vi "liveCameraView.vi"(1 "Data 16":u16[][](array[numeric])) -> (0 "VI Refnum":refnum<vi>)   [LabVIEW 2015]
panel:
  out "Image display":u16[][](graph)
  in  "Close window":bool
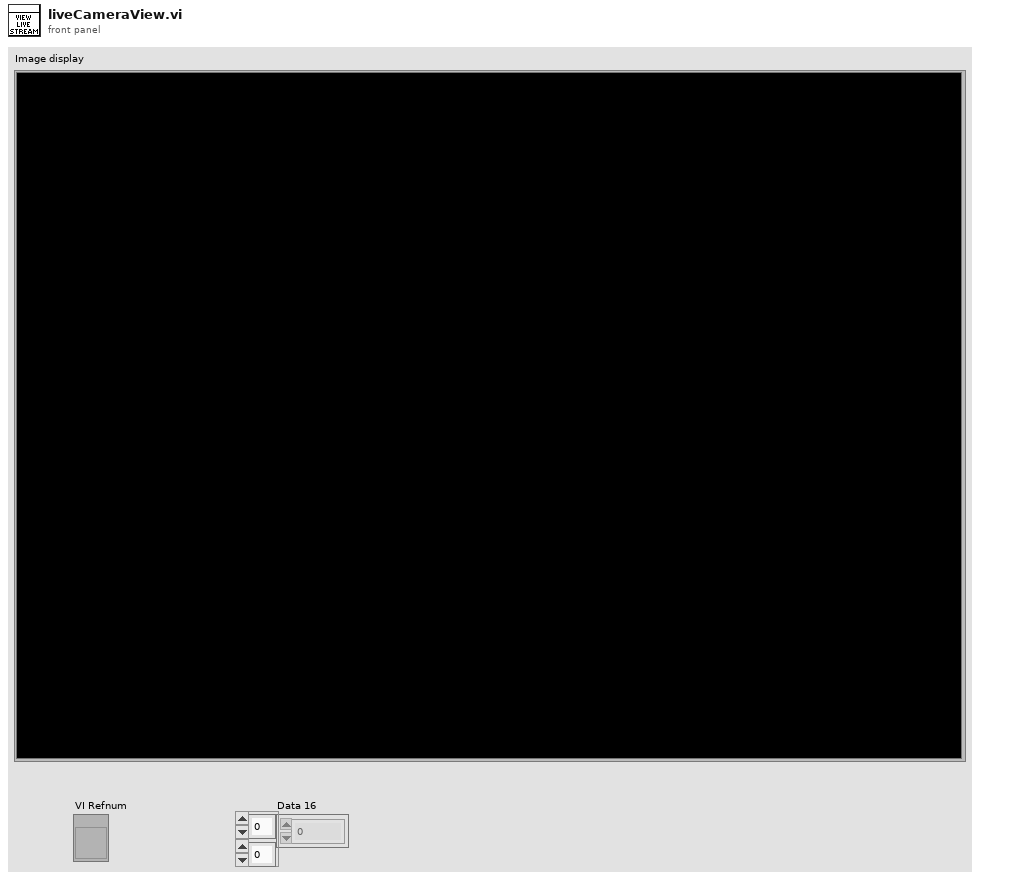
[diagram p1: front panel]
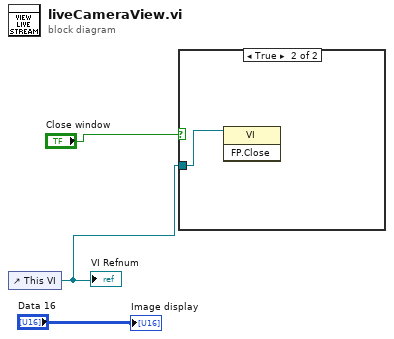
[diagram p0: block diagram]
diagram:
  n1 = control-ref of="This VI"() -> (w2:refnum<vi>)
  "VI Refnum" <- w2
  n2 = case shown="True" "Close window" {
    tunnel: w2 -> [_ w4]
    frame False {
    }
    frame True {
      n3 = invoke class="VI" method="FP.Close"(reference=w4) -> ()  [unwired: 2 in, 3 out]
    }
  }
  "Image display" <- "Data 16"
